vi "Accelerator Not Complex Graph.vi"(11 "nb_loop":i32=5) -> (3 "Model out":refnum<class "acc_Model.lvclass">)   [LabVIEW 2020]
uses:
  <vilib>/Graiphic/Accelerator/Source/Model/acc_Model.lvclass
  <vilib>/Graiphic/Accelerator/Source/Model/Controls/acc_input_parameters.ctl
  <vilib>/Graiphic/Accelerator/Source/Layer/Node/_Controls/acc_onnx_dtype_enum.ctl
  <vilib>/Graiphic/Accelerator/Source/Model/_Methods/add_to_graph/Initializer/acc_float_scalar_initializer.vi
  <vilib>/Graiphic/Accelerator/Source/Model/_Methods/add_to_graph/Numeric/acc_add_adaptive.vi
  <vilib>/Graiphic/Accelerator/Source/Model/_Methods/add_to_graph/Numeric/acc_mul_adaptive.vi
  <vilib>/Graiphic/Accelerator/Source/Model/_Methods/add_to_graph/Numeric/acc_div_adaptive.vi
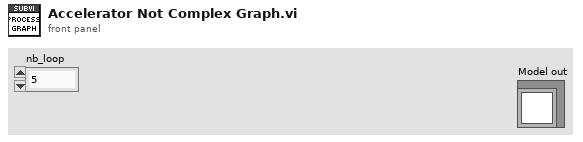
[diagram p1: front panel]
types:
  T1 = typedef "acc_input_parameters.ctl" = cluster{"Rank":enum16{"Scalar", "1D", "2D", "3D", "4D", "5D", "6D"}, "dtype":T2, "complex?":bool, "expert?":bool}
  T2 = typedef "acc_onnx_dtype_enum.ctl" = enum16{"UNDEFINED", "FLOAT", "UINT8", "INT8", "UINT16", "INT16", "INT32", "INT64", "STRING", "BOOL", "FLOAT16", "DOUBLE", "UINT32", "UINT64", "COMPLEX64", "COMPLEX128", "BFLOAT16", "FLOAT8E4M3FN", "FLOAT8E4M3FNUZ", "FLOAT8E5M2", "FLOAT8E5M2FNUZ", "UINT4", "INT4"}
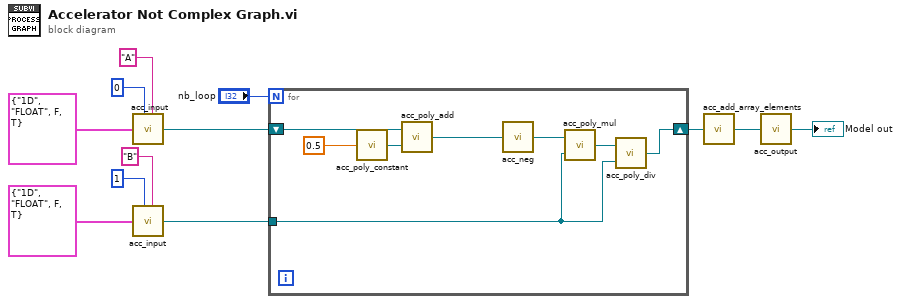
[diagram p0: block diagram]
diagram:
  n1 = call <vilib>:"acc_input.vi"("index"=0, "Parameters"=T1 {"Rank"=enum."1D", "dtype"=enum."FLOAT", "complex?"=FALSE, "expert?"=TRUE}, "input_name"="A") -> ("ONNXModel out"=w12:refnum<class "acc_Model.lvclass">)  [unwired: 6 in]
  n2 = call <vilib>:"acc_input.vi"("index"=1, "Parameters"=T1 {"Rank"=enum."1D", "dtype"=enum."FLOAT", "complex?"=FALSE, "expert?"=TRUE}, "input_name"="B") -> ("ONNXModel out"=w6:refnum<class "acc_Model.lvclass">)  [unwired: 6 in]
  n3 = for {
    N: "nb_loop" -> [_]
    tunnel: w6 -> [w14]
    shift-right: [w15] -> w5
    shift-left: w12 -> [w20]
    n4 = call-poly <vilib>:"acc_poly_constant.vi"("scalar"=sgl 0.5) -> ("Float Scalar"=w19:refnum<class "acc_Model.lvclass">)  [unwired: 3 in]
    n5 = call-poly <vilib>:"acc_poly_add.vi"("y"=w19, "x"=w20) -> ("x+y"=w13:refnum<class "acc_Model.lvclass">)
    n6 = call <vilib>:"acc_neg.vi"("x"=w13) -> ("-x"=w17:refnum<class "acc_Model.lvclass">)
    n7 = call-poly <vilib>:"acc_poly_mul.vi"("y"=w14, "x"=w17) -> ("x*y"=w16:refnum<class "acc_Model.lvclass">)
    n8 = call-poly <vilib>:"acc_poly_div.vi"("y"=w14, "x"=w16) -> ("x/y"=w15:refnum<class "acc_Model.lvclass">)
  }
  n9 = call <vilib>:"acc_add_array_elements.vi"("numeric array"=w5) -> ("sum"=w4:refnum<class "acc_Model.lvclass">)
  n10 = call <vilib>:"acc_output.vi"("ONNXModel in"=w4) -> ("ONNXModel out"=→"Model out":refnum<class "acc_Model.lvclass">)  [unwired: 8 in]
